vi "Create User.vi"(3 "error in (no error)":errorcluster, 4 "New user in":T1, 5 "Database.lvlib:Data Store.lvclass":refnum<class "Data Store.lvclass">) -> (0 "error out":errorcluster, 1 "UserID":i32, 2 "Database.lvlib:Data Store.lvclass 2":refnum<class "Data Store.lvclass">)   [LabVIEW 2011, in "Database.lvlib" / "Data Store.lvclass"]
uses:
  Data Store.lvclass
  User.ctl
  <vilib>/addons/database/Auxilliary.llb/DB Tools Transaction.ctl
  <vilib>/addons/database/Auxilliary.llb/DB Tools Isolation Level.ctl
  Data Store.lvclass/Data Store.ctl
  <vilib>/addons/database/Connection.llb/Conn Transaction.vi
  <vilib>/addons/database/Connection.llb/Conn Execute.vi
  <vilib>/addons/database/Recordset.llb/Rec Fetch Recordset Data (R).vi
  <vilib>/addons/database/Recordset.llb/Rec Destroy - Connection.vi
  <vilib>/addons/database/_DB Variant To Data/Database Variant To Data.xnode
  <vilib>/addons/database/NI_Database_API.lvlib
  Database.lvlib
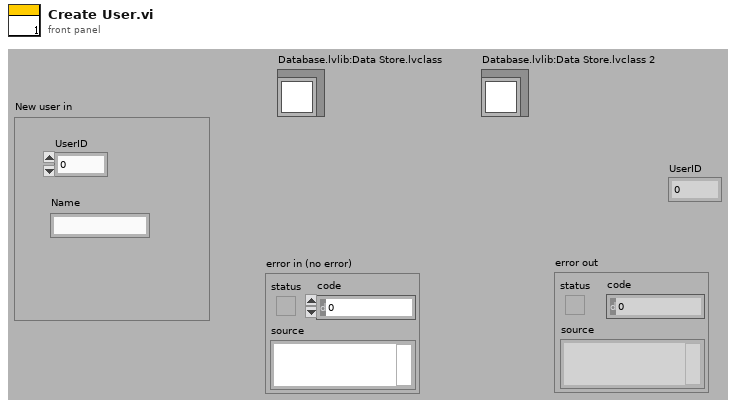
[diagram p1: front panel]
types:
  T1 = typedef "Database.lvlib/User.ctl" = cluster{"UserID":i32, "Name":string}
  T2 = typedef "NI_Database_API.lvlib/DB Tools Transaction.ctl" = enum16{"begin", "commit", "rollback"}
  T3 = typedef "NI_Database_API.lvlib/DB Tools Isolation Level.ctl" = enum16{"chaos", "read uncommitted", "read committed", "repeatable read", "serializable"}
  T4 = typedef "NI_Database_API.lvlib/Conn ObjectReference.ctl" = refnum<k1>
  T5 = typedef "NI_Database_API.lvlib/Rec ObjectReference.ctl" = refnum<k1>
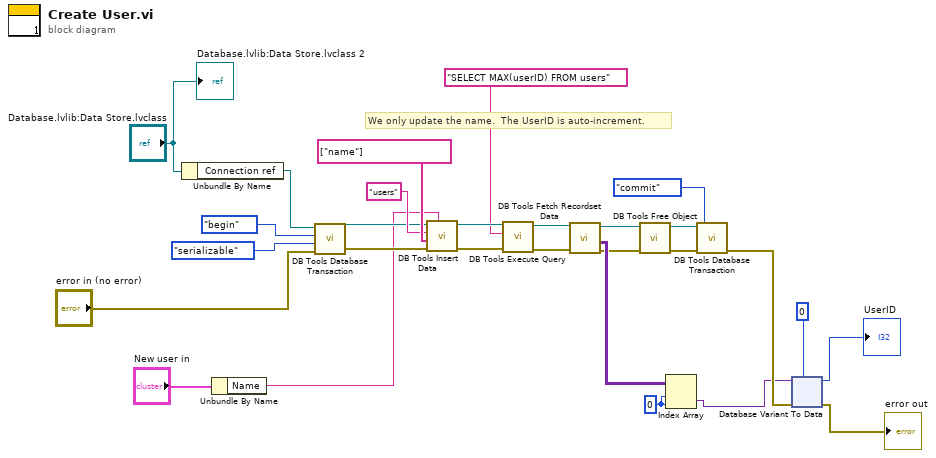
[diagram p0: block diagram]
diagram:
  w1 = 0 ("disabled index (col)")
  # "We only update the name.  The UserID is auto-increment."
  n1 = Unbundle By Name("Database.lvlib:Data Store.lvclass") -> ("Connection ref"=w27:T4)
  n2 = Unbundle By Name("New user in") -> ("Name"=w18:string)
  n3 = call-poly <vilib>:"DB Tools Database Transaction.vi"("error in (no error)"="error in (no error)", "isolation level (chaos)"=DB_Tools_Isolation_Level."serializable", "operation (begin)"=DB_Tools_Transaction."begin", "connection reference"=w27) -> ("error out"=w20:errorcluster, "connection reference out"=w21:T4)  [unwired: 2 in]
  n4 = call <vilib>:"DB Tools Insert Data.vi"("data"=w18, "error in (no error)"=w20, "columns"=string[] ["name"], "table"="users", "connection reference"=w21) -> ("error out"=w15:errorcluster, "connection reference out"=w17:T4)  [unwired: 5 in]
  n5 = call-poly <vilib>:"DB Tools Execute Query.vi"("error in (no error)"=w15, "SQL query"="SELECT MAX(userID) FROM users", "connection reference"=w17) -> ("error out"=w13:errorcluster, "recordset reference"=w14:T5)  [unwired: 5 in]
  n6 = call-poly <vilib>:"DB Tools Fetch Recordset Data.vi"("error in (no error)"=w13, "recordset reference"=w14) -> ("error out"=w9:errorcluster, "recordset data"=w12:variant[][], "recordset reference out"=w8:T5)  [unwired: 3 in]
  n7 = call-poly <vilib>:"DB Tools Free Object.vi"("error in (no error)"=w9, "recordset reference"=w8) -> ("error out"=w7:errorcluster, "connection reference"=w6:T4)  [unwired: 8 in]
  n8 = Index Array(array=w12, index (row)=w1, index (col)=w1) -> (element=w2:variant)
  n9 = call-poly <vilib>:"DB Tools Database Transaction.vi"("error in (no error)"=w7, "operation (begin)"=DB_Tools_Transaction."commit", "connection reference"=w6) -> ("error out"=w4:errorcluster)  [unwired: 3 in, 1 out]
  n10 = xnode "Database Variant To Data"("database variant"=w2, "error in"=w4, "type"=0 ("UserID")) -> ("data"=→"UserID":i32, "error out"=→"error out":errorcluster)
  "Database.lvlib:Data Store.lvclass 2" <- "Database.lvlib:Data Store.lvclass"
